vi "Select menu measurements.vi"(8 "error in (no error)":errorcluster, 10 "Measurements":string[](array[string]), 11 "Common Measurements Interface in":refnum<class "Common Measurements Interface.lvclass">) -> (0 "error out":errorcluster, 3 "Common Measurements Interface out":refnum<class "Common Measurements Interface.lvclass">)   [LabVIEW 2015, in "Common Measurements Interface.lvclass"]
uses:
  Common Measurements Interface.lvclass
  Common Measurements Interface.lvclass/Common Measurements Interface.ctl
  Queued Listbox/Queued Listbox.xctl
panel:
  out "Current value":string[](array[string])
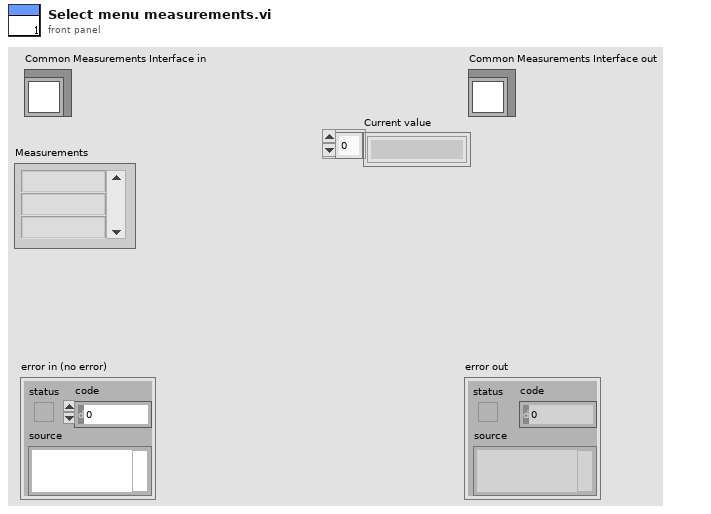
[diagram p1: front panel]
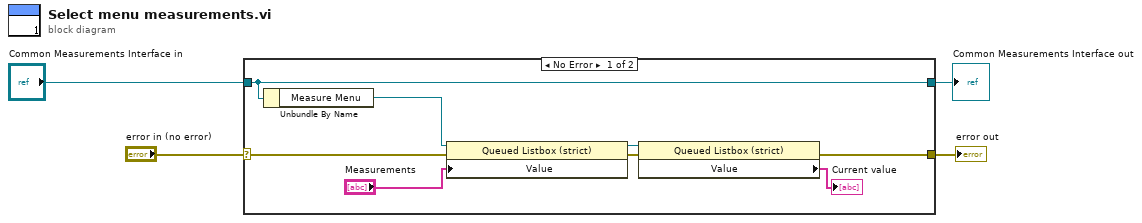
[diagram p0: block diagram]
diagram:
  n1 = case shown="No Error" "error in (no error)" {
    selector: "error in (no error)" -> [w9 w14]
    tunnel: [w6 w14] -> w3
    tunnel: [w12 w13] -> w1
    tunnel: "Common Measurements Interface in" -> [w12 w13]
    frame No Error {
      n2 = Unbundle By Name(w12) -> ("Measure Menu"=w11:refnum<vi>)
      n3 = property class="Queued Listbox (strict)"(reference=w11, error in=w9, "Value"="Measurements") -> (reference out=w8:refnum<vi>, error out=w7:errorcluster)
      n4 = property class="Queued Listbox (strict)"(reference=w8, error in=w7) -> (error out=w6:errorcluster, "Value"=→"Current value":string[])  [unwired: 1 out]
    }
    frame Error {
    }
  }
  "error out" <- w3
  "Common Measurements Interface out" <- w1
